vi "Config-Sender.vi"(8 "error in":errorcluster, 11 "Refnum in":T1) -> (0 "error out":errorcluster, 2 "Sender":T2, 3 "Refnum out":T1)   [LabVIEW 2021, in "UDP_Config.lvclass"]
uses:
  UDP_Config.lvclass
  Sender.ctl
  <vilib>/Utility/config.llb/Config Data RefNum.ctl
  <vilib>/Utility/config.llb/Read Key (U32).vi
  <vilib>/Utility/config.llb/NI_LVConfig.lvlib
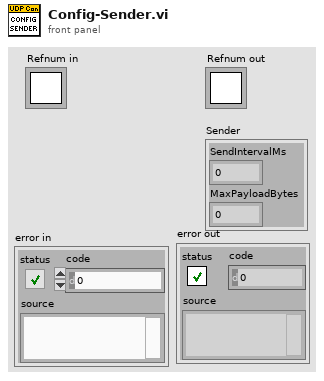
[diagram p1: front panel]
types:
  T1 = typedef "NI_LVConfig.lvlib/Config Data RefNum.ctl" = refnum<k1>
  T2 = typedef "Sender.ctl" = cluster{"SendIntervalMs":u32, "MaxPayloadBytes":u32}
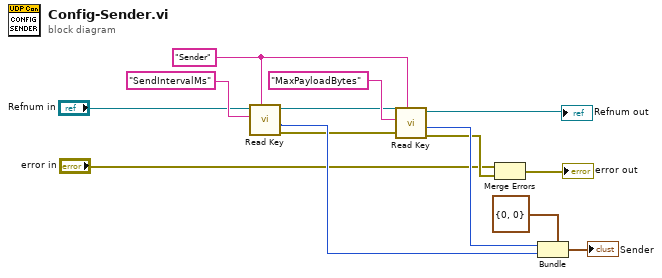
[diagram p0: block diagram]
diagram:
  w7 = "Sender" ("key")
  n1 = call-poly <vilib>:"Read Key.vi"("section"=w7, "key"="SendIntervalMs", "refnum"="Refnum in") -> ("error out"=w10:errorcluster, "value"=w11:u32, "refnum out"=w6:T1)  [unwired: 5 in, 1 out]
  n2 = call-poly <vilib>:"Read Key.vi"("section"=w7, "error in (no error)"=w10, "key"="MaxPayloadBytes", "refnum"=w6) -> ("error out"=w4:errorcluster, "value"=w12:u32, "refnum out"=→"Refnum out":T1)  [unwired: 4 in, 1 out]
  n3 = Merge Errors("error in", w4) -> (→"error out":errorcluster)
  n4 = Bundle(cluster=T2 {"SendIntervalMs"=0, "MaxPayloadBytes"=0} ("Sender"), "SendIntervalMs"=w12, "MaxPayloadBytes"=w11) -> (→"Sender":T2)
